vi "which_settings_to_save.vi"() -> (3 "Which settings to save 2":cluster{"Boolean":bool, "Setting":string}[](array[cluster])=[{"Boolean"=TRUE, "Setting"="Variables"}, {"Boolean"=TRUE, "Setting"="HSDIO"}, {"Boolean"=TRUE, "Setting"="DAQmx"}, {"Boolean"=TRUE, "Setting"="DDS"}, {"Boolean"=TRUE, "Setting"="Camera"}, {"Boolean"=TRUE, "Setting"="Counters"}, {"Boolean"=TRUE, "Setting"="Filters"}, {"Boolean"=TRUE, "Setting"="AnalogOutput"}, {"Boolean"=TRUE, "Setting"="Notes"}, {"Boolean"=TRUE, "Setting"="GPIB"}, {"Boolean"=TRUE, "Setting"="PhysikInstrumentePiezo"}, {"Boolean"=TRUE, "Setting"="Andor"}] caption="Choose which settings to save:")   [LabVIEW 2013]
doc: "MTL 2012-12-24\n\nThis VI give allows the user to choose which of the settings will be save into a config file. This allows for flexibility for combining settings from several experiments."
panel:
  in  "Which settings to save":cluster{"Boolean":bool, "Setting":string}[](array[cluster])=[{"Boolean"=TRUE, "Setting"="Variables"}, {"Boolean"=TRUE, "Setting"="HSDIO"}, {"Boolean"=TRUE, "Setting"="DAQmx"}, {"Boolean"=TRUE, "Setting"="DDS"}, {"Boolean"=TRUE, "Setting"="Camera"}, {"Boolean"=TRUE, "Setting"="Counters"}, {"Boolean"=TRUE, "Setting"="Filters"}, {"Boolean"=TRUE, "Setting"="AnalogOutput"}, {"Boolean"=TRUE, "Setting"="Notes"}, {"Boolean"=TRUE, "Setting"="GPIB"}, {"Boolean"=TRUE, "Setting"="PhysikInstrumentePiezo"}, {"Boolean"=TRUE, "Setting"="Andor"}] caption="Choose which settings to save:"
  in  "Boolean":bool
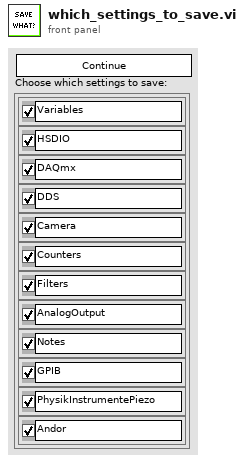
[diagram p1: front panel]
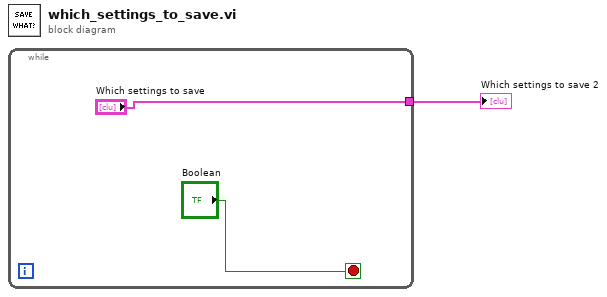
[diagram p0: block diagram]
diagram:
  n1 = while {
    tunnel: ["Which settings to save"] -> w1
    stop <- "Boolean" stop-if-true
  }
  "Which settings to save 2" <- w1
